vi "serialize.vi"() -> ()   [LabVIEW 2013, in "async tests.lvlib"]
uses:
  async tests.lvlib
  configuration/asynchronous execution module configuration.lvclass
  tests/test module/module/configuration/TEST CONFIGURATION.lvclass
  configuration/asynchronous execution module configuration.lvclass/asynchronous execution module configuration.ctl
  configuration/Write contained configuration.vi
  configuration/Write execution period (ms).vi
  <vilib>/NI/Tag Bus Module Framework/root configuration/TBM configuration.lvclass
panel:
  out "no error":errorcluster
  out "OK":bool
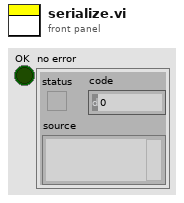
[diagram p1: front panel]
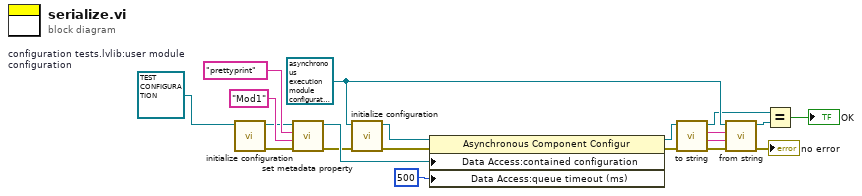
[diagram p0: block diagram]
diagram:
  w1 = refnum<class "TEST CONFIGURATION.lvclass"> refnum  # configuration tests.lvlib:user module configuration
  w10 = refnum<class "asynchronous execution module configuration.lvclass"> refnum ("Asynchronous Component Configuration")
  n1 = call-dynamic "initialize configuration.vi"("configuration in"=w1) -> ("error out"=w4:errorcluster, "configuration out"=w11:refnum<class "TEST CONFIGURATION.lvclass">)  [unwired: 8 in, 1 out]
  n2 = call <vilib>:"set metadata property.vi"("error in"=w4, "value"="Mod1" ("format string"), "key"="prettyprint", "configuration in"=w11) -> ("error out"=w3:errorcluster, "configuration out"=w19:refnum<class "TEST CONFIGURATION.lvclass">)  [unwired: 6 in]
  n3 = call-dynamic "initialize configuration.vi"("error in"=w3, "configuration in"=w10) -> ("error out"=w2:errorcluster, "configuration out"=w9:refnum<class "asynchronous execution module configuration.lvclass">)  [unwired: 7 in, 1 out]
  n4 = property class="Asynchronous Component Configur"(reference=w9, error in=w2, "Data Access:contained configuration"=w19, "Data Access:queue timeout (ms)"=500 ("queue timeout (ms)")) -> (reference out=w15:refnum<class "asynchronous execution module configuration.lvclass">, error out=w16:errorcluster)
  n5 = call-dynamic "to string.vi"("error in"=w16, "asynchronous execution module configuration In"=w15) -> ("error out"=w14:errorcluster, "data"=w12:string, "version"=w13:string, "asynchronous execution module configuration Out"=w7:refnum<class "asynchronous execution module configuration.lvclass">)  [unwired: 6 in]
  n6 = call-dynamic "from string.vi"("error in"=w14, "data"=w12, "version"=w13, "asynchronous execution module configuration In"=w10) -> ("error out"=→"no error":errorcluster, "asynchronous execution module configuration Out"=w8:refnum<class "asynchronous execution module configuration.lvclass">)  [unwired: 6 in]
  n7 = Equal?(x=w7, y=w8) -> (x = y?=→"OK":bool)
